vi "LAN.vi"() -> ()   [LabVIEW 2012]
panel:
  in  "タイムアウト":u32=10
  in  "終了ボタン":bool
  in  "クリアボタン":bool
  in  "送受信ボタン":bool
  out "受信文字列":string
  in  "コマンド":string="*IDN?"
  in  "ポート番号":string="3500"
  in  "IPアドレス":string="192.168.0.1"
  # "秒"
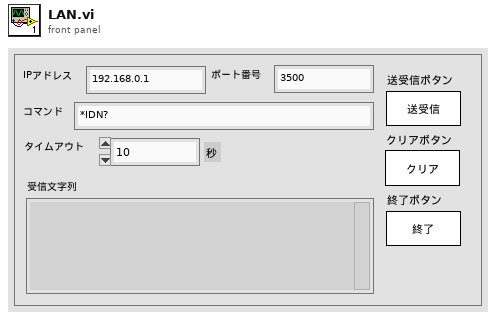
[diagram p1: front panel]
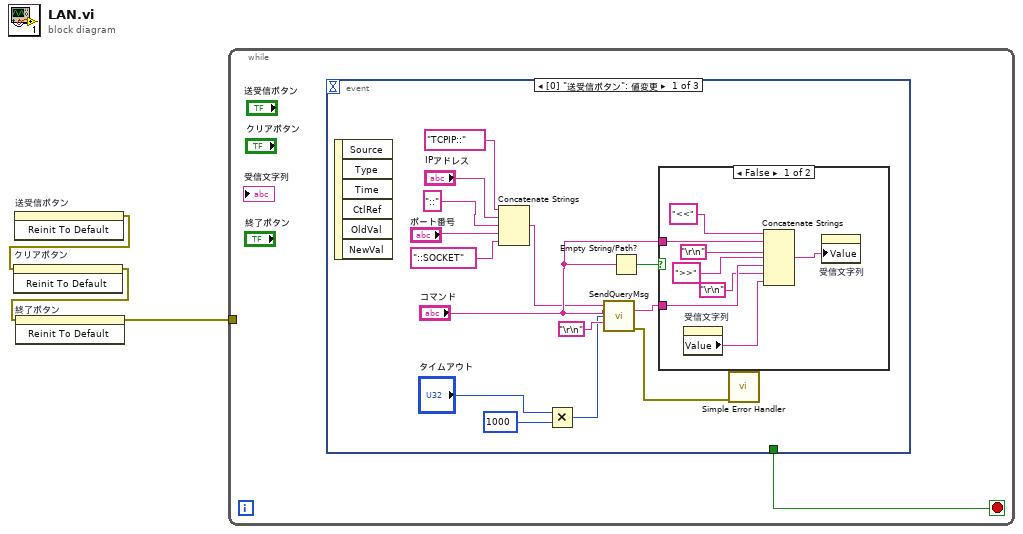
[diagram p0: block diagram]
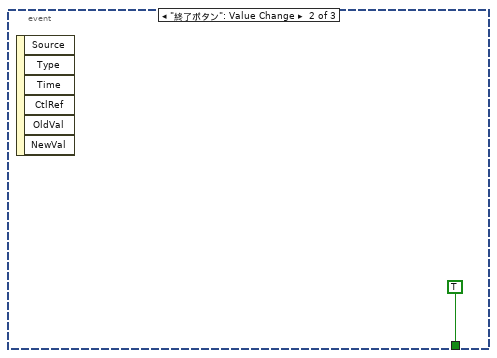
[diagram p3: hidden frame]
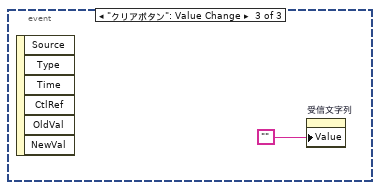
[diagram p4: hidden frame]
diagram:
  n1 = invoke on="送受信ボタン" class="Bool" method="Reinit To Default"() -> (error out=w3:errorcluster)  [unwired: 3 in, 2 out]
  n2 = invoke on="クリアボタン" class="Bool" method="Reinit To Default"(error in=w3) -> (error out=w2:errorcluster)  [unwired: 2 in, 2 out]
  n3 = invoke on="終了ボタン" class="Bool" method="Reinit To Default"(error in=w2) -> (error out=w1:errorcluster)  [unwired: 2 in, 2 out]
  n4 = while {
    tunnel: w1 -> [_]
    stop <- w4 stop-if-true
    n5 = event shown="[0] \"送受信ボタン\": 値変更" {
      selector: _ -> [_ _ _]
      dyn-events: _ -> [_ _ _]
      timeout: _ -> [_ _ _]
      tunnel: [_ TRUE _] -> w4
      event "送受信ボタン": Value Change {
        n6 = event-data() -> ()  [unwired: 1 in, 6 out]
        n7 = Concatenate Strings("TCPIP::", "IPアドレス", "::", "ポート番号", "::SOCKET") -> (w9:string)
        n8 = Multiply(x="タイムアウト", y=u32 1000) -> (x*y=w6:u32)
        n9 = call "SendQueryMsg.vi"("VISAリソース名"=w9, "入力文字列"="コマンド", "タイムアウト"=w6, "ターミネータ"="\r\n") -> ("受信文字列"=w12:string, "エラー出力"=w11:errorcluster)  [unwired: 10 in]
        n10 = Empty String/Path?(string/path="コマンド") -> (empty?=w13:bool)
        n11 = case shown="FALSE" w13 {
          tunnel: w12 -> [w21 _]
          tunnel: "コマンド" -> [w24 _]
          frame False {
            n12 = property on="受信文字列" class="Str"() -> ("Value"=w19:string)  [unwired: 2 in, 2 out]
            n13 = Concatenate Strings("<<", w24, "\r\n", ">>", w21, "\r\n", w19) -> (w26:string)
            n14 = property on="受信文字列" class="Str"("Value"=w26) -> ()  [unwired: 2 in, 2 out]
          }
          frame True {
          }
        }
        n15 = call <vilib>:"Simple Error Handler.vi"("error in (no error)"=w11) -> ()  [unwired: 4 in, 5 out]
      }
      event "終了ボタン": Value Change {
        n16 = event-data() -> ()  [unwired: 1 in, 6 out]
      }
      event "クリアボタン": Value Change {
        n17 = event-data() -> ()  [unwired: 1 in, 6 out]
        n18 = property on="受信文字列" class="Str"("Value"="") -> ()  [unwired: 2 in, 2 out]
      }
    }
  }
